vi "verify operation mode.vi"(8 "error in (no error)":errorcluster, 11 "Channel in":refnum<class "Channel.lvclass">) -> (0 "error out":errorcluster, 3 "Channel out":refnum<class "Channel.lvclass">)   [LabVIEW 2018, in "Channel.lvclass"]
uses:
  Channel.lvclass
  Channel.lvclass/Channel.ctl
  Sim_CCD/Sim_CCD.lvclass/Sim_CCD.ctl
  Sim_CCD/Sim_CCD.lvclass
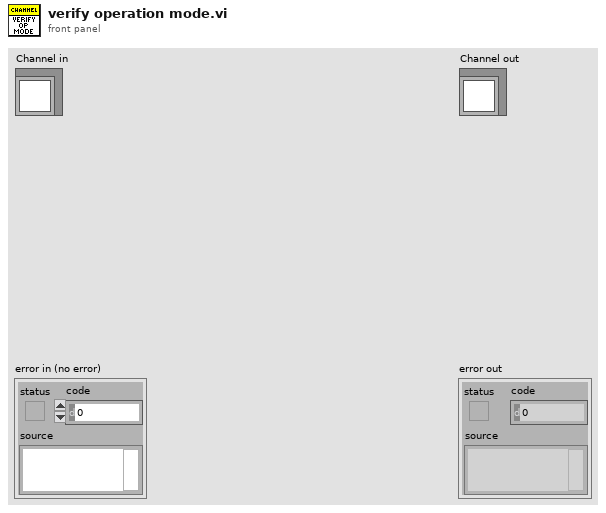
[diagram p1: front panel]
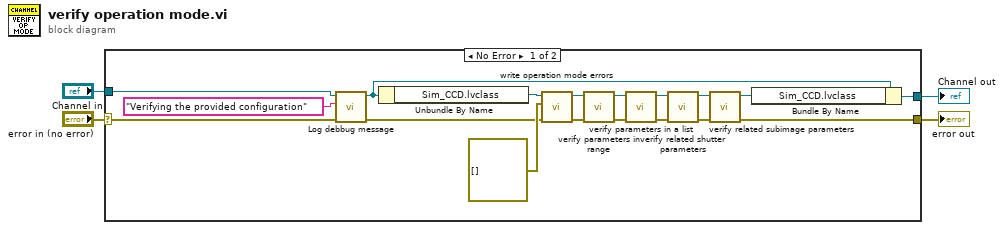
[diagram p0: block diagram]
diagram:
  n1 = case shown="No Error" "error in (no error)" {
    selector: "error in (no error)" -> [w16 w24]
    tunnel: [w5 w24] -> w3
    tunnel: [w6 w23] -> w1
    tunnel: "Channel in" -> [w18 w23]
    frame No Error {
      n2 = call "Log debbug message.vi"("error in (no error)"=w16, "String"="Verifying the provided configuration", "Channel in"=w18) -> ("error out"=w17:errorcluster, "Channel out"=w8:refnum<class "Channel.lvclass">)  [unwired: 7 in]
      n3 = Unbundle By Name(w8) -> ("Sim_CCD.lvclass"=w20:refnum<class "Sim_CCD.lvclass">)
      n4 = call "write operation mode errors.vi"("error in (no error)"=w17, "WRITE SETUP errors"=errorcluster[] [] ("Errors array"), "Simulated_CCD_Camera in"=w20) -> ("error out"=w21:errorcluster, "Simulated_CCD_Camera out"=w22:refnum<class "Sim_CCD.lvclass">)  [unwired: 7 in]
      n5 = call-dynamic "verify parameters in range.vi"("error in (no error)"=w21, "Simulated_CCD_Camera in"=w22) -> ("error out"=w12:errorcluster, "Simulated_CCD_Camera out"=w11:refnum<class "Sim_CCD.lvclass">)  [unwired: 8 in]
      n6 = call-dynamic "verify parameters in a list.vi"("error in (no error)"=w12, "Simulated_CCD_Camera in"=w11) -> ("error out"=w10:errorcluster, "Simulated_CCD_Camera out"=w9:refnum<class "Sim_CCD.lvclass">)  [unwired: 8 in]
      n7 = call "verify related shutter parameters.vi"("error in (no error)"=w10, "Simulated_CCD_Camera in"=w9) -> ("error out"=w13:errorcluster, "Simulated_CCD_Camera out"=w14:refnum<class "Sim_CCD.lvclass">)  [unwired: 8 in]
      n8 = call "verify related subimage parameters.vi"("error in (no error)"=w13, "Simulated_CCD_Camera in"=w14) -> ("error out"=w5:errorcluster, "Simulated_CCD_Camera out"=w7:refnum<class "Sim_CCD.lvclass">)  [unwired: 8 in]
      n9 = Bundle By Name(cluster=w8, "Sim_CCD.lvclass"=w7) -> (w6:refnum<class "Channel.lvclass">)
    }
    frame Error {
    }
  }
  "error out" <- w3
  "Channel out" <- w1
